vi "Example.vi"() -> ()   [LabVIEW 2013, in "QWTBLVLib.lvlib"]
doc: "Clears Matlab variables, set working path, writes input data, writes calculation settings, calls algorithm, reads output data."
uses:
  QWTBLVLib.lvlib
  TD Quantity.ctl
  TD Calculation Settings.ctl
  TD Uncertainty Calculation Method.ctl
  TD Correlation Calculation Settings.ctl
  TD DOF Calculation Settings.ctl
  TD MCM Calculation Settings.ctl
  TD MCM Calculation Method.ctl
panel:
  in  "QWTB Folder Path:":path=path "C:/Data/qwtb/qwtb"
  in  "Amplitude":dbl=1.2345
  in  "Phase (deg)":dbl=12.345 caption="Phase"
  in  "Frequency":dbl=1.12345
  out "ph (rad)":dbl[][](array[numeric])
  out "A":dbl[][](array[numeric])
  out "f":dbl[][](array[numeric])
  out "error out":errorcluster
  # "Example for QWTBLVLib\n1, Set path to QWTB folder.\n2, Run vi.\nA sine waveform will be generated and PSFE algorithm\nwill be used to calculate waveform parameters"
  # "Set Waveform parameters:"
  # "Calculated waveform parameters:"
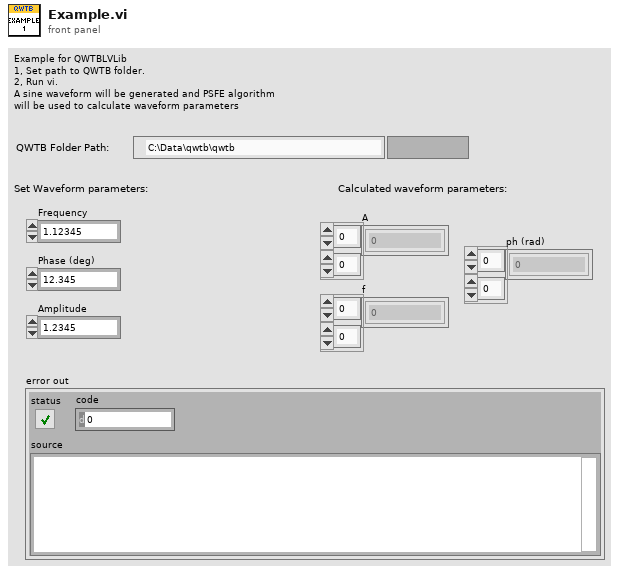
[diagram p1: front panel]
types:
  T1 = typedef "QWTBLVLib.lvlib/TD Quantity.ctl" = cluster{"Name":string, "Value":dbl[][], "Uncertainty":dbl[][], "Degrees of Freedom":dbl[][], "Correlation":dbl[][], "Randomized uncertainty":dbl[][]}
  T2 = typedef "QWTBLVLib.lvlib/TD Calculation Settings.ctl" = cluster{"Strict":bool, "Verbose":bool, "Uncertainty Calculation Method":T3, "Correlations":T4, "Degrees of Freedom":T5, "MCM Calculation Settings":T6}
  T3 = typedef "QWTBLVLib.lvlib/TD Uncertainty Calculation Method.ctl" = enum16{"none", "GUF", "MCM"}
  T4 = typedef "QWTBLVLib.lvlib/TD Correlation Calculation Settings.ctl" = cluster{"Required":bool, "Generate":bool}
  T5 = typedef "QWTBLVLib.lvlib/TD DOF Calculation Settings.ctl" = cluster{"Required":bool, "Generate":bool}
  T6 = typedef "QWTBLVLib.lvlib/TD MCM Calculation Settings.ctl" = cluster{"Repeats":i32, "Verbose":bool, "Parallelization method":T7, "Processors":i32, "Temporary directory":string, "Randomize":bool}
  T7 = typedef "QWTBLVLib.lvlib/TD MCM Calculation Method.ctl" = enum16{"Single Core", "Multi Core", "Multi Station"}
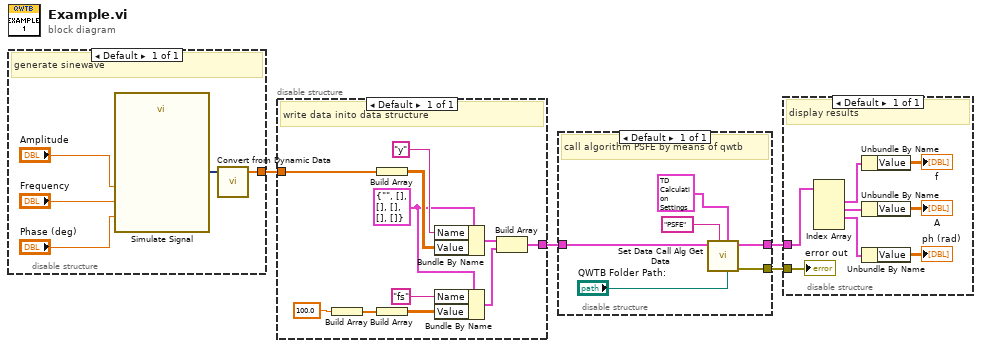
[diagram p0: block diagram]
diagram:
  n1 = disable-structure shown="Default" {
    disable-tunnel: [w5] -> w1
    frame Enabled {
      # "generate sinewave"
      n2 = call "Simulate Signal"("Frequency"="Frequency", "Amplitude"="Amplitude", "Phase"="Phase (deg)") -> ("Sine"=w6:dynamicdata)  [unwired: 11 in, 1 out]
      n3 = call "Convert from Dynamic Data"("Dynamic Data Type"=w6) -> ("Array"=w5:dbl[])  [unwired: 3 in]
    }
  }
  n4 = disable-structure shown="Default" {
    disable-tunnel: [w17] -> w4
    disable-tunnel: w1 -> [w10]
    frame Enabled {
      w16 = T1 {"Name"="", "Value"=[], "Uncertainty"=[], "Degrees of Freedom"=[], "Correlation"=[], "Randomized uncertainty"=[]} ("Quantity")
      # "write data inito data structure"
      n5 = Build Array(100.0 ("Numeric")) -> (w12:dbl[])
      n6 = Build Array(w10) -> (w20:dbl[][])
      n7 = Build Array(w12) -> (w11:dbl[][])
      n8 = Bundle By Name(cluster=w16, "Name"="y", "Value"=w20) -> (w18:T1)
      n9 = Bundle By Name(cluster=w16, "Name"="fs", "Value"=w11) -> (w15:T1)
      n10 = Build Array(w18, w15) -> (w17:T1[])
    }
  }
  n11 = disable-structure shown="Default" {
    disable-tunnel: w4 -> [w24]
    disable-tunnel: [w23] -> w3
    disable-tunnel: [w21] -> w2
    frame Enabled {
      # "call algorithm PSFE by means of qwtb"
      n12 = call "Set Data Call Alg Get Data.vi"("QWTB Folder Path"="QWTB Folder Path:", "Calculation Settings"=T2 {"Strict"=FALSE, "Verbose"=TRUE, "Uncertainty Calculation Method"=enum."none", "Correlations"={"Required"=FALSE, "Generate"=FALSE}, "Degrees of Freedom"={"Required"=FALSE, "Generate"=FALSE}, "MCM Calculation Settings"={"Repeats"=100, "Verbose"=TRUE, "Parallelization method"=enum."Single Core", "Processors"=1, "Temporary directory"=".", "Randomize"=TRUE}}, "Algorithm ID"="PSFE", "Data In"=w24) -> ("error out"=w23:errorcluster, "Data Out"=w21:T1[])  [unwired: 6 in]
    }
  }
  n13 = disable-structure shown="Default" {
    disable-tunnel: w3 -> [w34]
    disable-tunnel: w2 -> [w33]
    frame Enabled {
      # "display results"
      n14 = Index Array(array=w33) -> (element #1=w32:T1, element #2=w31:T1, element #3=w30:T1)  [unwired: 4 in, 1 out]
      n15 = Unbundle By Name(w32) -> ("Value"=→"f":dbl[][])
      n16 = Unbundle By Name(w31) -> ("Value"=→"A":dbl[][])
      n17 = Unbundle By Name(w30) -> ("Value"=→"ph (rad)":dbl[][])
      "error out" <- w34
    }
  }
